vi "FTW-Actor-HandleSubscriberMessages.vi"(0 "FTW-ActorInstance In":refnum<class "FTW-ActorInstance.lvclass">, 5 "FTW Incoming Request In":refnum<class "FTW-Message.lvclass">, 11 "error in":errorcluster) -> (4 "FTW-ActorInstance Out":refnum<class "FTW-ActorInstance.lvclass">, 15 "error out":errorcluster)   [LabVIEW 2015, in "FTW-ActorInstance.lvclass"]
uses:
  FTW-ActorInstance.lvclass
  Message/Base/FTW-Message.lvclass
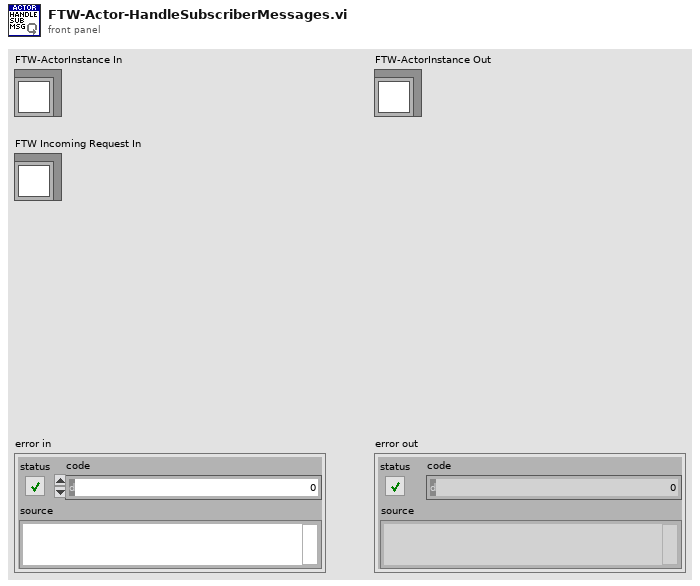
[diagram p1: front panel]
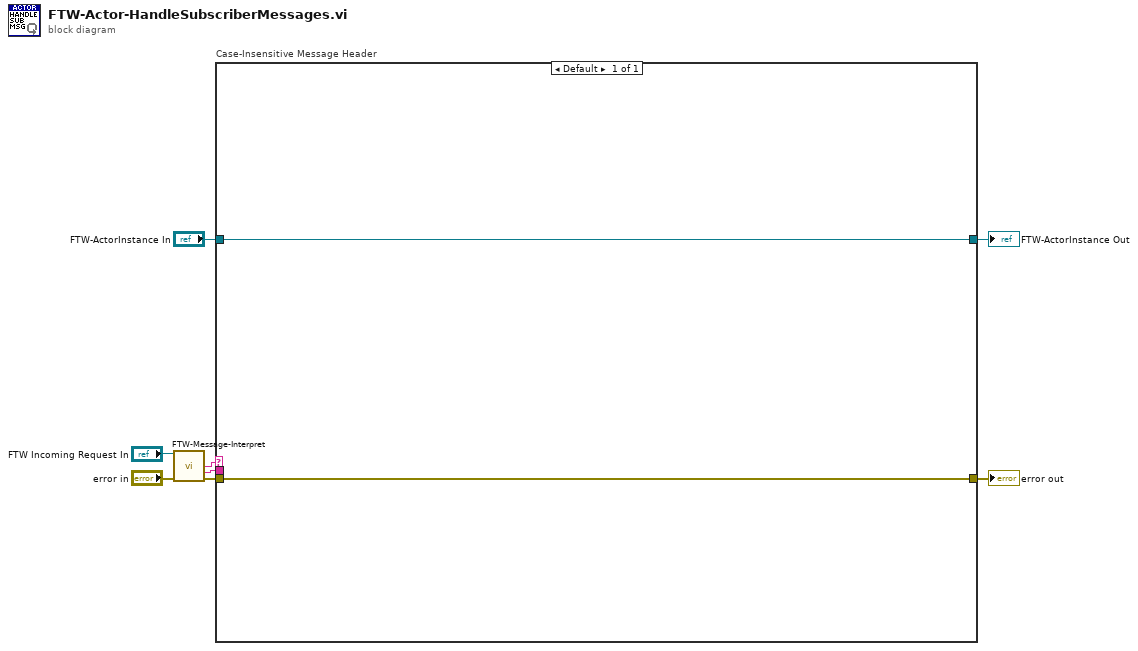
[diagram p0: block diagram]
diagram:
  n1 = call-dynamic "FTW-Message-Interpret.vi"("FTW Message"="FTW Incoming Request In", "error in"="error in") -> ("Message Header"=w1:string, "Message Body"=w7:string, "error out"=w8:errorcluster)  [unwired: 9 in, 2 out]
  n2 = case "Case-Insensitive Message Header" shown="Default" w1 {
    tunnel: [w9] -> w2
    tunnel: w8 -> [w9]
    tunnel: [w10] -> w3
    tunnel: "FTW-ActorInstance In" -> [w10]
    tunnel: w7 -> [_]
    frame Default {
    }
  }
  "FTW-ActorInstance Out" <- w3
  "error out" <- w2
